vi "Grids0008.vi"   [LabVIEW 2013]
uses:
  <vilib>/Heliosphere Research LLC/Advanced Plotting Toolkit/api_core/NewPlotScales.ctl
  <vilib>/Heliosphere Research LLC/Advanced Plotting Toolkit/Advanced Plotting Toolkit.lvlib
types:
  T1 = typedef "Advanced Plotting Toolkit.lvlib/NewPlotScales.ctl" = enum16{"Default", "Linear", "Log", "Symlog"}
  T2 = typedef "Advanced Plotting Toolkit.lvlib/PlotID.ctl" = i32
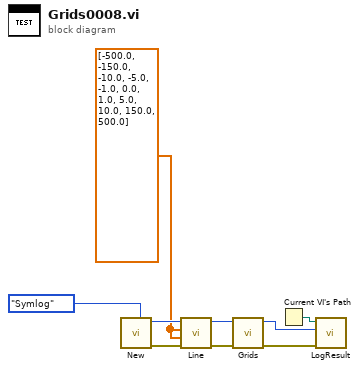
[diagram p0: block diagram]
diagram:
  w5 = dbl[] [-500.0, -150.0, -10.0, -5.0, -1.0, 0.0, 1.0, 5.0, 10.0, 150.0, 500.0] ("X Data")
  n1 = call <vilib>:"New.vi"("Y Axis Scale"=NewPlotScales."Symlog") -> ("error out"=w4:errorcluster, "Plot ID"=w6:T2)  [unwired: 9 in]
  n2 = call <vilib>:"Line.vi"("error in (no error)"=w4, "Y Data"=w5, "X Data"=w5, "Plot ID"=w6) -> ("error out"=w1:errorcluster, "Plot ID out"=w2:T2)  [unwired: 6 in]
  n3 = call <vilib>:"Grids.vi"("error in (no error)"=w1, "Plot ID"=w2) -> ("error out"=w7:errorcluster, "Plot ID Out"=w8:T2)  [unwired: 8 in]
  n4 = Current VI's Path() -> (path=w9:path)
  n5 = call "LogResult.vi"("Test Result"=w7, "Test Artifact"=w8, "VI Path"=w9) -> ()  [unwired: 9 in]
